vi "RunControl.vi"(8 "error in (no error)":errorcluster, 11 "PTC10":T1={"serial settings"={"port"="Stanford_PTC10", "baud rate"=9600}, "PTC10 Info"={"Manufacturer"="", "Instrument"="", "Serial Number"="", "Firmware"=""}, "VISA resource name"="", "pwmloop"="define pwmloop(#t=0 while (1) {waitforsample if(#pwm=0){relays=0}else{if(#t<#pwm) {relays=1}else{relays=3}}#t+=1 if  (#t>99){#t=0} pause 0.2 s})", "onecycle"="define onecycle (pwm=100 run pwmloop 5A.PID.Setpoint=-130.0 5A.PID.input=3C while(#3C>-129.0){pause 0.2 s}pwm=-130 pause 10 min pwm=0  5A.PID.SetPoint=50.0 while(#3C<49.0){pause 0.2 s} pause 10 min kill pwmloop)", "control"="define control (#count=1 while (#count>=0) {onecycle pause 1 s #count-=1})", "HeatDrive"="define Failsafe (while(1) {if (#Check <-20){relays=0 outputEnable Off}else{if(#Check>20){relays=0 outputEnable Off}} pause 1 s})", "ToAmbient"="define ToAmbient(if(#3C>25.0){pwm=100 run pwmloop while(#3C>#25.0){pause 0.5 s} pwm=0 kill pwmloop}else{#5A.PID.setpoint=20.0 while(#3C<15.0){pause 0.5 s} outputenable off})", "StartupCode"="system.display.Monitors Show", "LogChannels"=[], "Heater O/P Channel"="", " Control Input"="", "TAmbient"=20.0, "AmbientTolerance"=5.0, "TestCycleParameters"={"TAmb"=20.0, "HeaterTestTemp"=20.0, "HeaterTestDwell(min)"=1, "HeaterTestDuration"=1, "MinOpTemp"=-131.5, "MinOpDwell(min)"=30, "TestHeatingRate (deg/min)"=0.4, "SurviveCycleParameters"={"MinSurviveTemp"=-131.5, "MinSurvive Dwell(min)"=10, "MaxSurviveTemp"=50.0, "MaxSurviveDwell(min)"=30, "ControlInput"=2, "ColdStandOff"=4.0, "HotStandoff"=5.0, "SteadyPWM"=20, "MaxCoolingRate (deg/min)"=3.75, "MaxHeatingRate (deg/min)"=2.5}, "CycleType"=0, "MaxOpTemp"=-50.0, "MaxOpDwell(min)"=30}, "PID Params"={"P"=1.14, "I"=0.012, "D"=21.68, "Set"=0.0}} {"PID Params"."D" min=0.0; "PID Params"."I" min=0.0; "PID Params"."P" min=0.0; "TestCycleParameters"."CycleType" items=["Survival", "Operational"]; "TestCycleParameters"."SurviveCycleParameters"."SteadyPWM" min=0 max=100 step=1; "TestCycleParameters"."SurviveCycleParameters"."ControlInput" items=["3A", "3B", "3C", "3D", "4A", "4B", "4C", "4D"]; "serial settings"."baud rate" items=["9600"=9600, "19200"=19200, "38400"=38400, "57600"=57600, "115200"=115200]}) -> (0 "error out":errorcluster, 3 "PTC10 2":T1={"serial settings"={"port"="Stanford_PTC10", "baud rate"=9600}, "PTC10 Info"={"Manufacturer"="", "Instrument"="", "Serial Number"="", "Firmware"=""}, "VISA resource name"="", "pwmloop"="define pwmloop(#t=0 while (1) {waitforsample if(#pwm=0){relays=0}else{if(#t<#pwm) {relays=1}else{relays=3}}#t+=1 if  (#t>99){#t=0} pause 0.2 s})", "onecycle"="define onecycle (pwm=100 run pwmloop 5A.PID.Setpoint=-130.0 5A.PID.input=3C while(#3C>-129.0){pause 0.2 s}pwm=-130 pause 10 min pwm=0  5A.PID.SetPoint=50.0 while(#3C<49.0){pause 0.2 s} pause 10 min kill pwmloop)", "control"="define control (#count=1 while (#count>=0) {onecycle pause 1 s #count-=1})", "HeatDrive"="define Failsafe (while(1) {if (#Check <-20){relays=0 outputEnable Off}else{if(#Check>20){relays=0 outputEnable Off}} pause 1 s})", "ToAmbient"="define ToAmbient(if(#3C>25.0){pwm=100 run pwmloop while(#3C>#25.0){pause 0.5 s} pwm=0 kill pwmloop}else{#5A.PID.setpoint=20.0 while(#3C<15.0){pause 0.5 s} outputenable off})", "StartupCode"="system.display.Monitors Show", "LogChannels"=[], "Heater O/P Channel"="", " Control Input"="", "TAmbient"=20.0, "AmbientTolerance"=5.0, "TestCycleParameters"={"TAmb"=20.0, "HeaterTestTemp"=20.0, "HeaterTestDwell(min)"=1, "HeaterTestDuration"=1, "MinOpTemp"=-131.5, "MinOpDwell(min)"=30, "TestHeatingRate (deg/min)"=0.4, "SurviveCycleParameters"={"MinSurviveTemp"=-131.5, "MinSurvive Dwell(min)"=10, "MaxSurviveTemp"=50.0, "MaxSurviveDwell(min)"=30, "ControlInput"=2, "ColdStandOff"=4.0, "HotStandoff"=5.0, "SteadyPWM"=20, "MaxCoolingRate (deg/min)"=3.75, "MaxHeatingRate (deg/min)"=2.5}, "CycleType"=0, "MaxOpTemp"=-50.0, "MaxOpDwell(min)"=30}, "PID Params"={"P"=1.14, "I"=0.012, "D"=21.68, "Set"=0.0}} {"PID Params"."D" min=0.0; "PID Params"."I" min=0.0; "PID Params"."P" min=0.0; "TestCycleParameters"."CycleType" items=["Survival", "Operational"]; "TestCycleParameters"."SurviveCycleParameters"."SteadyPWM" min=0 max=100 step=1; "TestCycleParameters"."SurviveCycleParameters"."ControlInput" items=["3A", "3B", "3C", "3D", "4A", "4B", "4C", "4D"]; "serial settings"."baud rate" items=["9600"=9600, "19200"=19200, "38400"=38400, "57600"=57600, "115200"=115200]})   [LabVIEW 2024]
uses:
  controls/SRS PTC10.ctl
  controls/TestCycleParams.ctl
  controls/SurviveCycleParams.ctl
  controls/ControlInput.ctl
  controls/PID Params.ctl
  <instrlib>/Stanford PTC10/SRS PTC10.lvlib
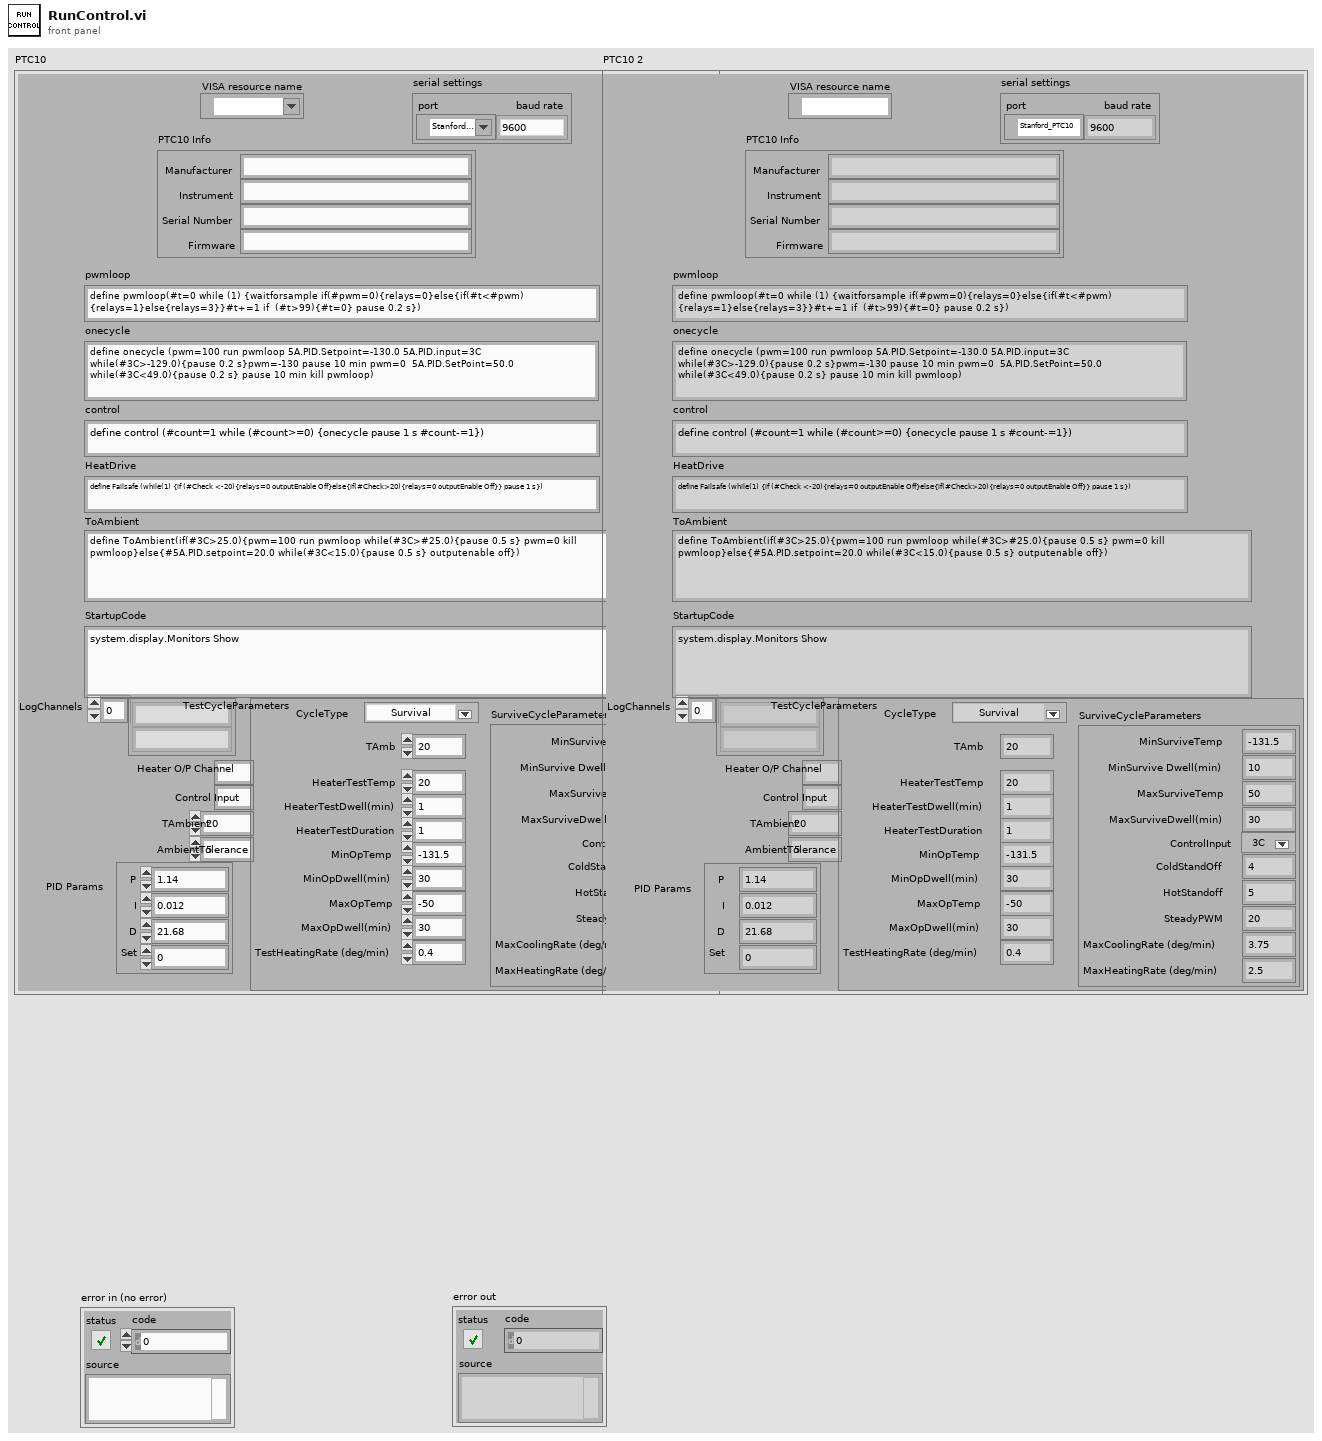
[diagram p1: front panel]
types:
  T1 = typedef "SRS PTC10.ctl" = cluster{"serial settings":cluster{"port":refnum<visa-resource-name>, "baud rate":u32}, "PTC10 Info":cluster{"Manufacturer":string, "Instrument":string, "Serial Number":string, "Firmware":string}, "VISA resource name":refnum<visa-resource-name>, "pwmloop":string, "onecycle":string, "control":string, "HeatDrive":string, "ToAmbient":string, "StartupCode":string, "LogChannels":string[], "Heater O/P Channel":string, " Control Input":string, "TAmbient":dbl, "AmbientTolerance":dbl, "TestCycleParameters":T2, "PID Params":T5}
  T2 = typedef "TestCycleParams.ctl" = cluster{"TAmb":dbl, "HeaterTestTemp":dbl, "HeaterTestDwell(min)":i32, "HeaterTestDuration":i32, "MinOpTemp":dbl, "MinOpDwell(min)":i32, "TestHeatingRate (deg/min)":dbl, "SurviveCycleParameters":T3, "CycleType":u16, "MaxOpTemp":dbl, "MaxOpDwell(min)":i32}
  T3 = typedef "SurviveCycleParams.ctl" = cluster{"MinSurviveTemp":dbl, "MinSurvive Dwell(min)":i32, "MaxSurviveTemp":dbl, "MaxSurviveDwell(min)":i32, "ControlInput":T4, "ColdStandOff":dbl, "HotStandoff":dbl, "SteadyPWM":i32, "MaxCoolingRate (deg/min)":dbl, "MaxHeatingRate (deg/min)":dbl}
  T4 = typedef "ControlInput.ctl" = u16
  T5 = typedef "PID Params.ctl" = cluster{"P":dbl, "I":dbl, "D":dbl, "Set":dbl}
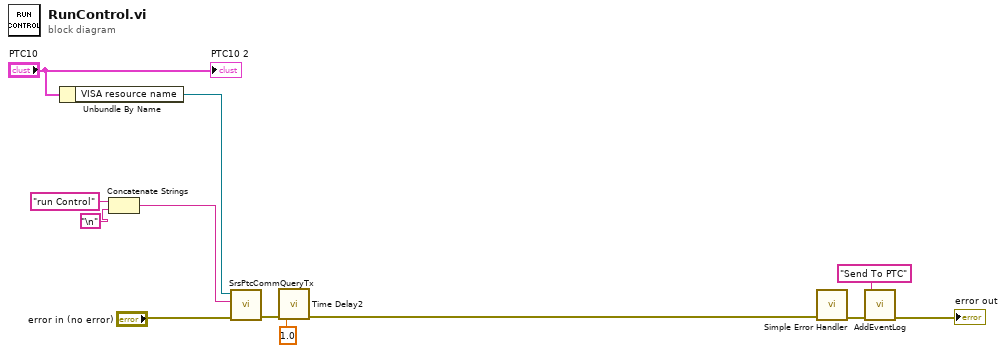
[diagram p0: block diagram]
diagram:
  n1 = Unbundle By Name("PTC10") -> ("VISA resource name"=w6:refnum<visa-resource-name>)
  n2 = Concatenate Strings("run Control" ("string"), "\n") -> (w2:string)
  n3 = call <instrlib>:"SrsPtcCommQueryTx.vi"("error in"="error in (no error)", "Query"=w2, "SRS PTC10 VISA in"=w6) -> ("error out"=w10:errorcluster)  [unwired: 6 in, 2 out]
  n4 = call "Time Delay2"("error in (no error)"=w10, "Delay Time (s)"=1.0) -> ("error out"=w5:errorcluster)  [unwired: 9 in]
  n5 = call <vilib>:"Simple Error Handler.vi"("error in (no error)"=w5) -> ("error out"=w12:errorcluster)  [unwired: 4 in, 4 out]
  n6 = call "AddEventLog.vi"("error in (no error)"=w12, "Event"="Send To PTC") -> ("error out"=→"error out":errorcluster)  [unwired: 9 in]
  "PTC10 2" <- "PTC10"
